vi "EndTestCase.vi"(7 "Time":dbl format="%#_13g", 8 "error in (no error)":errorcluster, 10 "Test":refnum<class "Test.lvclass">, 11 "TestResult in":refnum<class "TestResult.lvclass">) -> (0 "error out":errorcluster, 3 "TestResult out":refnum<class "TestResult.lvclass">)   [LabVIEW 2017, in "TestResult.lvclass"]
uses:
  TestResult.lvclass
  TestListener/TestListener.lvclass
  Test/Test.lvclass
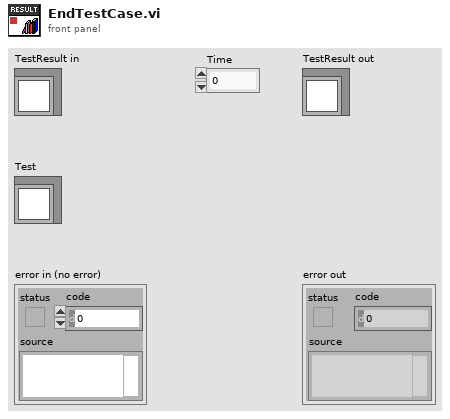
[diagram p1: front panel]
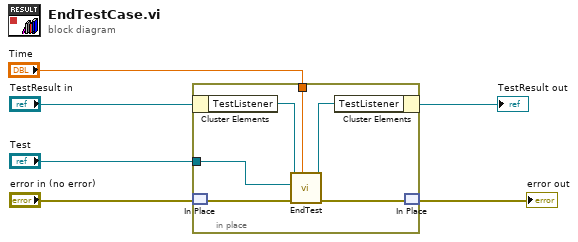
[diagram p0: block diagram]
diagram:
  n1 = in-place {
    in-place-border: "Test" -> [w12]
    in-place-border: "Time" -> [w7]
    n2 = in-place-cluster #1("TestResult in") -> ("TestListener"=w9:refnum<class "TestListener.lvclass">)
    n3 = in-place-match #2("error in (no error)") -> (w11:errorcluster)
    n4 = call-dynamic "EndTest.vi"("Time"=w7, "error in (no error)"=w11, "Test"=w12, "TestListener in"=w9) -> ("error out"=w10:errorcluster, "TestListener out"=w8:refnum<class "TestListener.lvclass">)  [unwired: 6 in]
    n5 = in-place-cluster #1("TestListener"=w8) -> (→"TestResult out":refnum<class "TestResult.lvclass">)
    n6 = in-place-match #2(w10) -> (→"error out":errorcluster)
  }
